vi "uploadBinImage.vi"(6 "binFile":path, 7 "dloadAddr":u32 format="%.0x", 8 "Error in":errorcluster {"code" format="%.0x"}, 11 "canSession":T1) -> (0 "Error out":errorcluster {"code" format="%.0x"}, 1 "msgData":T2[](array[typedef]) {"Data" format="%.0x"; "ArbitrationId" format="%.0x"; "Timestamp" format="%<%I:%M:%S%3u %p\n%m/%d/%Y>T"}, 3 "canSession":T1)   [LabVIEW 2017]
doc: "Demonstrates how to write and receive CAN frames via the Network Interface on the same port. \n\nTo write and receive frames via the Network Interface:\n- select the CAN Network Interface (i.e. CAN0, CAN1, etc.)\n- select the Baud Rate\n- run the VI\n- press the write button to write frames to the can bus\n\nEnable RTR Button to send a Remote Transmission Request or to simply send an empty Frame to request an Answer Frame from a connected device.\n\nEnable Extended Button to write extended Identifier Format. This is done by setting the 30th bit to enable extended format with the driver."
uses:
  <vilib>/nican/nican.llb/CanFrameTimed.ctl
  <vilib>/nican/nican.llb/xobjhandle.ctl
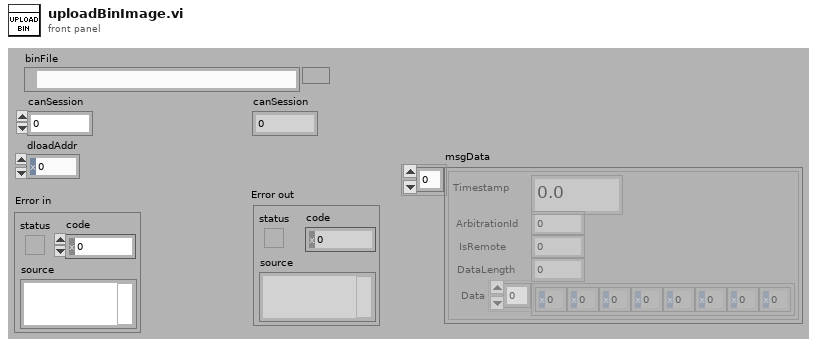
[diagram p1: front panel]
types:
  T1 = typedef "xobjhandle.ctl" = u32
  T2 = typedef "CanFrameTimed.ctl" = cluster{"Timestamp":dbl, "ArbitrationId":u32, "IsRemote":u8, "DataLength":u8, "Data":u8[]}
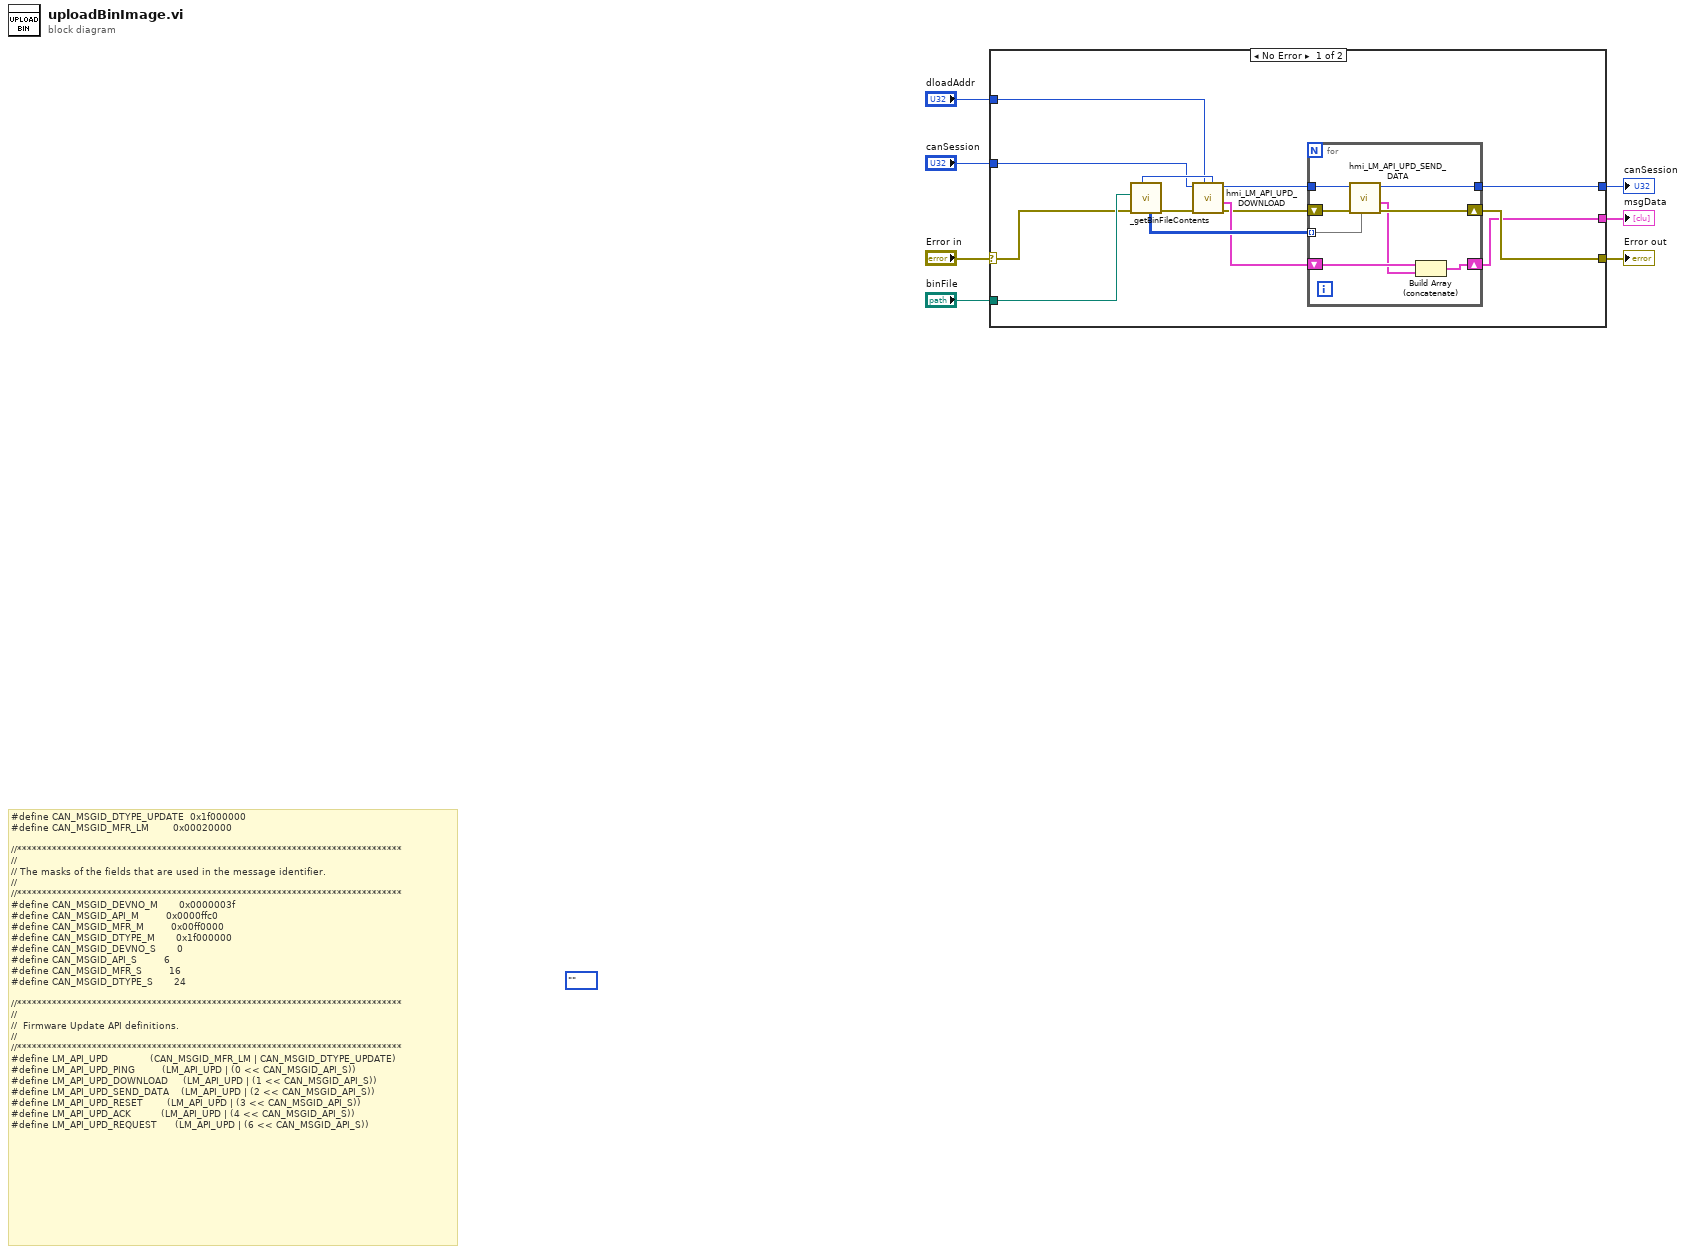
[diagram p0: block diagram]
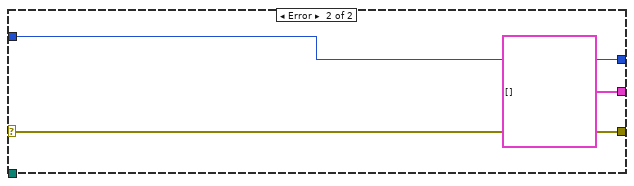
[diagram p2: hidden frame]
diagram:
  (unwired) enum32{""}.""
  # "#define CAN_MSGID_DTYPE_UPDATE  0x1f000000\n#define CAN_MSGID_MFR_LM        0x00020000\n\n//*****************************************************************************\n//\n// The masks of the fields that are used in the message identifier.\n//\n//*****************************************************************************\n#define CAN_MSGID_DEVNO_M       0x0000003f\n#define CAN_MSGID_API_M         0x0000ffc0\n#define CAN_MSGID_MFR_M         0x00ff0000\n#define CAN_MSGID_DTYPE_M       0x1f000000\n#define CAN_MSGID_DEVNO_S       0\n#define CAN_MSGID_API_S         6\n#define CAN_MSGID_MFR_S         16\n#define CAN_MSGID_DTYPE_S       24\n\n//*****************************************************************************\n//\n//  Firmware Update API definitions.\n//\n//*****************************************************************************\n#define LM_API_UPD              (CAN_MSGID_MFR_LM | CAN_MSGID_DTYPE_UPDATE)\n#define LM_API_UPD_PING         (LM_API_UPD | (0 << CAN_MSGID_API_S))\n#define LM_API_UPD_DOWNLOAD     (LM_API_UPD | (1 << CAN_MSGID_API_S))\n#define LM_API_UPD_SEND_DATA    (LM_API_UPD | (2 << CAN_MSGID_API_S))\n#define LM_API_UPD_RESET        (LM_API_UPD | (3 << CAN_MSGID_API_S))\n#define LM_API_UPD_ACK          (LM_API_UPD | (4 << CAN_MSGID_API_S))\n#define LM_API_UPD_REQUEST      (LM_API_UPD | (6 << CAN_MSGID_API_S))"
  n1 = case shown="No Error" "Error in" {
    selector: "Error in" -> [w13 w31]
    tunnel: [w14 T2[] [] ("msgData")] -> w7
    tunnel: "canSession" -> [w9 w30]
    tunnel: [w19 w30] -> w5
    tunnel: [w20 w31] -> w4
    tunnel: "dloadAddr" -> [w10 _]
    tunnel: "binFile" -> [w16 _]
    frame No Error {
      n2 = call "_getBinFileContents.vi"("error in"=w13, "binFile"=w16) -> ("error out"=w12:errorcluster, "chunkedData"=w17:u8[][], "numBytes"=w11:i64)  [unwired: 5 in, 2 out]
      n3 = call "hmi_LM_API_UPD_DOWNLOAD.vi"("dloadSize"=w11, "dloadAddr"=w10, "Error in"=w12, "canSession"=w9) -> ("Error out"=w8:errorcluster, "msgData"=w15:T2[], "canSession"=w18:T1)  [unwired: 5 in]
      n4 = for {
        shift-right: [w28] -> w20
        shift-left: w8 -> [w25]
        tunnel: w18 -> [w26]
        tunnel: [w27] -> w19
        tunnel: w17 -> [w24] mode=indexing
        shift-right: [w22] -> w14
        shift-left: w15 -> [w23]
        n5 = call "hmi_LM_API_UPD_SEND_DATA.vi"("data"=w24, "Error in"=w25, "canSession"=w26) -> ("Error out"=w28:errorcluster, "msgData"=w21:T2[], "canSession"=w27:T1)  [unwired: 6 in]
        n6 = Build Array (concatenate)(w23, w21) -> (w22:T2[])
      }
    }
    frame Error {
    }
  }
  "msgData" <- w7
  "canSession" <- w5
  "Error out" <- w4
